vi "HEWH RLT Update Station Channel Control.vi"(7 "Unit":T2, 8 "Error In":errorcluster, 9 "TC Channels":string[](array[string])=["011", "013", "015", "017", "019", "020"], 10 "Panel In":T1[][](array[typedef]), 11 "Station In":T3) -> (0 "Error Out":errorcluster, 2 "Panel Out":T1[][](array[typedef]), 3 "Station Out":T3)   [LabVIEW 2016]
uses:
  Custom Instrument Control/MW100/Type Definitions/Station ID Selector.ctl
  Type Definitions/HEWH RLT Stations.ctl
  Type Definitions/HEWH Label Channel.ctl
  Type Definitions/HEWH Channel Label RLT.ctl
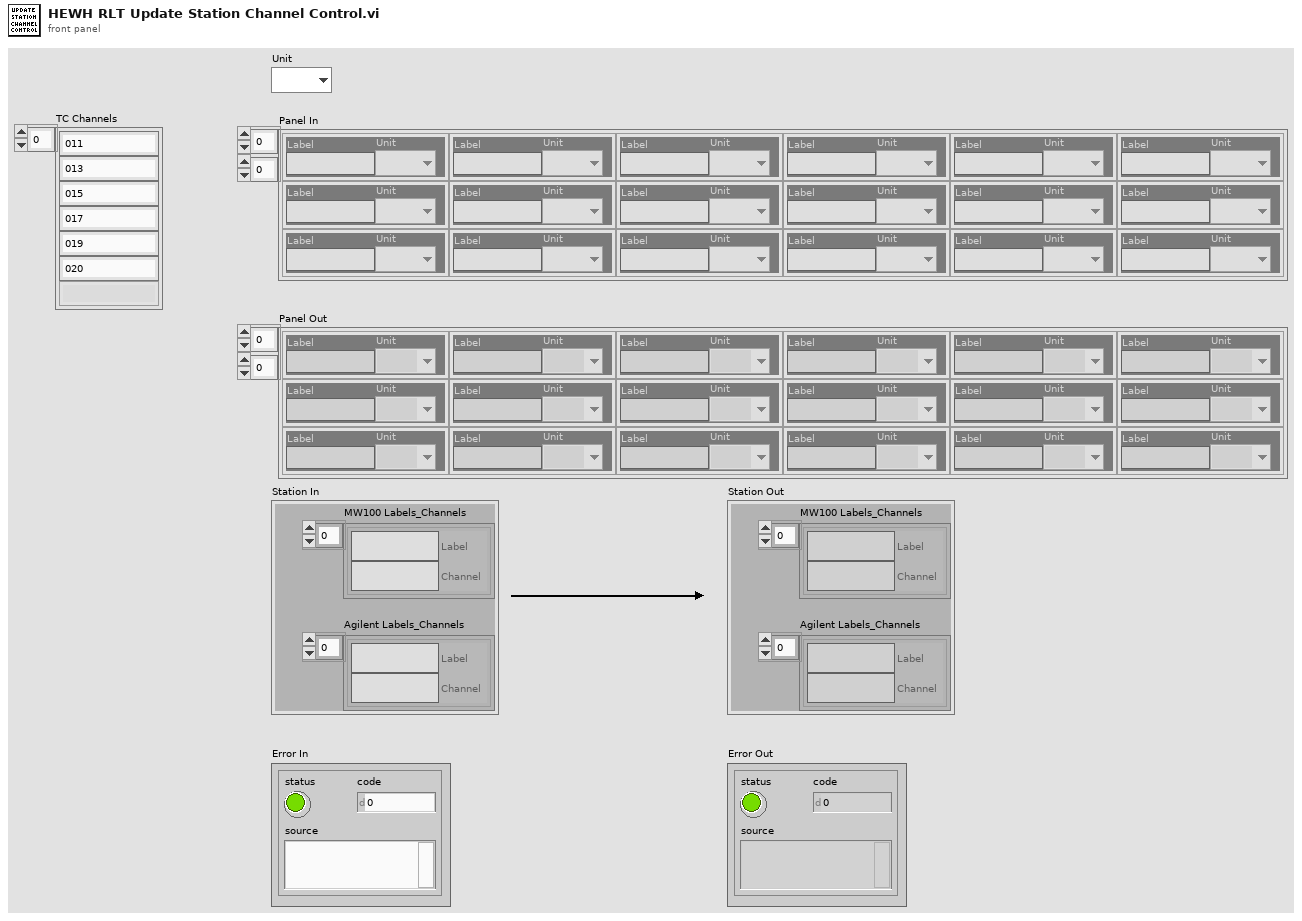
[diagram p1: front panel]
types:
  T1 = typedef "HEWH Channel Label RLT.ctl" = cluster{"Label":string, "Unit":T2}
  T2 = typedef "Station ID Selector.ctl" = enum16{"", "A", "B", "C", "D", "Global"}
  T3 = typedef "HEWH RLT Stations.ctl" = cluster{"MW100 Labels_Channels":T4[], "Agilent Labels_Channels":T4[]}
  T4 = typedef "HEWH Label Channel.ctl" = cluster{"Label":string, "Channel":string}
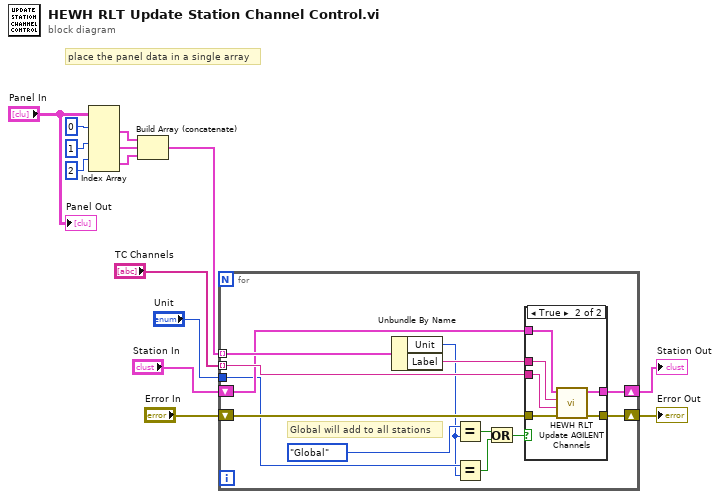
[diagram p0: block diagram]
diagram:
  # "place the panel data in a single array"
  n1 = Index Array(array="Panel In", index (row) #1=0 ("index (row)"), index (row) #2=1 ("index (row)"), index (row) #3=2 ("index (row)")) -> (element #1=w8:T1[], element #2=w9:T1[], element #3=w10:T1[])  [unwired: 3 in]
  n2 = Build Array (concatenate)(w8, w9, w10) -> (w13:T1[])
  n3 = for {
    tunnel: w13 -> [w27] mode=indexing
    tunnel: "TC Channels" -> [w26] mode=indexing
    shift-right: [w23] -> w12
    shift-left: "Station In" -> [w24]
    tunnel: "Unit" -> [w19]
    shift-right: [w21] -> w3
    shift-left: "Error In" -> [w22]
    # "Global will add to all stations"
    n4 = Unbundle By Name(w27) -> ("Unit"=w15:T2, "Label"=w25:string)
    n5 = Equal?(x=Station_ID_Selector."Global" ("y"), y=w15) -> (x = y?=w18:bool)
    n6 = Equal?(x=w19, y=w15) -> (x = y?=w17:bool)
    n7 = Or(x=w18, y=w17) -> (x .or. y?=w16:bool)
    n8 = case shown="True" w16 {
      tunnel: w26 -> [_ w33]
      tunnel: w25 -> [_ w32]
      tunnel: w24 -> [w29 w35]
      tunnel: [w29 w34] -> w23
      tunnel: w22 -> [w28 w31]
      tunnel: [w28 w30] -> w21
      frame False {
      }
      frame True {
        n9 = call "HEWH RLT Update AGILENT Channels.vi"("Error In"=w31, "Channel"=w33, "Label"=w32, "Station A in"=w35) -> ("Error Out"=w30:errorcluster, "Station A out"=w34:T3)  [unwired: 6 in]
      }
    }
  }
  "Station Out" <- w12
  "Error Out" <- w3
  "Panel Out" <- "Panel In"
